vi "PD_Control.vi"() -> ()   [LabVIEW 2017]
uses:
  <vilib>/Platform/TimedLoop/XDataNode/timing_clust.ctl
  <vilib>/Platform/TimedLoop/XDataNode/nitl_modes.ctl
  <vilib>/Platform/TimedLoop/XDataNode/wakeup.ctl
  <vilib>/myRIO/Instrument Drivers/Onboard IO/AO/typedefs/AO Reference.ctl
  <vilib>/myRIO/Common/Instrument Driver Framework/Utilities/typedefs/myRIO Generic Hardware Reference.ctl
  <vilib>/myRIO/Common/Instrument Driver Framework/Utilities/typedefs/Hardware Version Enum.ctl
  <vilib>/myRIO/Common/Instrument Driver Framework/Utilities/typedefs/myRIO v1.0 Reference.ctl
  <vilib>/myRIO/Common/Instrument Driver Framework/Utilities/typedefs/Generic FPGA Reference.ctl
  <vilib>/myRIO/Common/Instrument Driver Framework/myRIO v1.0/AO/typedefs/AO Channels List.ctl
  <vilib>/myRIO/Common/Instrument Driver Framework/myRIO v1.0/AO/typedefs/AO Channels Enum.ctl
  <vilib>/myRIO/Common/Instrument Driver Framework/Utilities/typedefs/Analog Scaling Constants List.ctl
  <vilib>/myRIO/Common/Instrument Driver Framework/Utilities/typedefs/Analog Scaling Constants.ctl
  <vilib>/userdefined/High Color/nirio_resource_hc.ctl
  <vilib>/myRIO/Common/Instrument Driver Framework/Utilities/vis/Is FPGA Ref Available.vi
  <vilib>/myRIO/Common/Instrument Driver Framework/myRIO v1.0/AO/vis/myRIO v1.1 Open AO.vi
  <vilib>/myRIO/Instrument Drivers/Onboard IO/AO/vis/Write.vi
  <vilib>/myRIO/Common/Instrument Driver Framework/Utilities/vis/Validate Channels.vi
  <vilib>/myRIO/Common/Instrument Driver Framework/myRIO v1.0/AO/vis/myRIO v1.0 Reserve AO.vi
  <vilib>/myRIO/Common/Instrument Driver Framework/myRIO v1.0/AO/vis/myRIO v1.0 Build MUX Configuration AO.vi
  <vilib>/myRIO/Common/Instrument Driver Framework/myRIO v1.0/Resource Manager/vis/myRIO v1.0 Reserve Channel List.vi
  <vilib>/myRIO/Common/Instrument Driver Framework/myRIO v1.0/Resource Manager/vis/myRIO v1.0 Reserve Channel.vi
  <vilib>/myRIO/Common/Instrument Driver Framework/myRIO v1.0/Resource Manager/vis/myRIO v1.0 Unreserve Channel.vi
  <vilib>/myRIO/Common/Instrument Driver Framework/myRIO v1.0/Resource Manager/vis/myRIO v1.0 Build Mutex Name.vi
  <vilib>/Utility/VariantDataType/GetNumericInfo.vi
  <vilib>/Utility/error.llb/Error Cluster From Error Code.vi
  <vilib>/myRIO/Common/Instrument Driver Framework/myRIO v1.0/myRIO v1.1 Open.vi
  <vilib>/myRIO/Common/Instrument Driver Framework/myRIO v1.0/AO/vis/myRIO v1.0 Get Scaling Constants AO.vi
  <vilib>/myRIO/Common/Instrument Driver Framework/Utilities/vis/IO Manager.vi
  <vilib>/myRIO/Common/Instrument Driver Framework/Utilities/vis/Configuration Manager.vi
  <vilib>/myRIO/Common/Instrument Driver Framework/myRIO v1.0/myRIO v1.0 Close.vi
  <vilib>/myRIO/Common/Instrument Driver Framework/myRIO v1.0/AO/vis/myRIO v1.0 Write AO.vi
  <vilib>/addons/control/pid/pid.llb/PID (DBL).vi
  <vilib>/platform/TimedLoop/XDataNode/XDataNode.xnode
  <vilib>/myRIO/Express VI/Onboard IO/AO/AO Express VI.xnode
  <vilib>/myRIO/Instrument Drivers/Onboard IO/AO/vis/myRIO AO Open.xnode
  <vilib>/addons/control/pid/NI_PID_pid.lvlib
  <vilib>/myRIO/Instrument Drivers/Onboard IO/AO/AO.lvlib
  <vilib>/Platform/TimedLoop/XDataNode/XDNodeRunTimeDep.lvlib
panel:
  out "error out":errorcluster
  out "process variable":dbl
  out "Setpoint":dbl
  out "Analog Output":dbl(graph)=3.193359702
  out "output":dbl format="%.2f"
  in  "PID Range":cluster{"output high":dbl, "output low":dbl}={"output high"=3.2, "output low"=1.8} {"output low" format="%.2f"; "output high" format="%.2f"}
  in  "PID gains":T1={"proportional gain (Kc)"=2.0, "integral time (Ti, min)"=0.05, "derivative time (Td, min)"=0.0} {"derivative time (Td, min)" format="%.3f"; "integral time (Ti, min)" format="%.3f"; "proportional gain (Kc)" format="%.3f"}
  out "Distance":cluster{"setpoint":dbl, dbl}(graph)={"setpoint"=303.908879655711, 0.0}
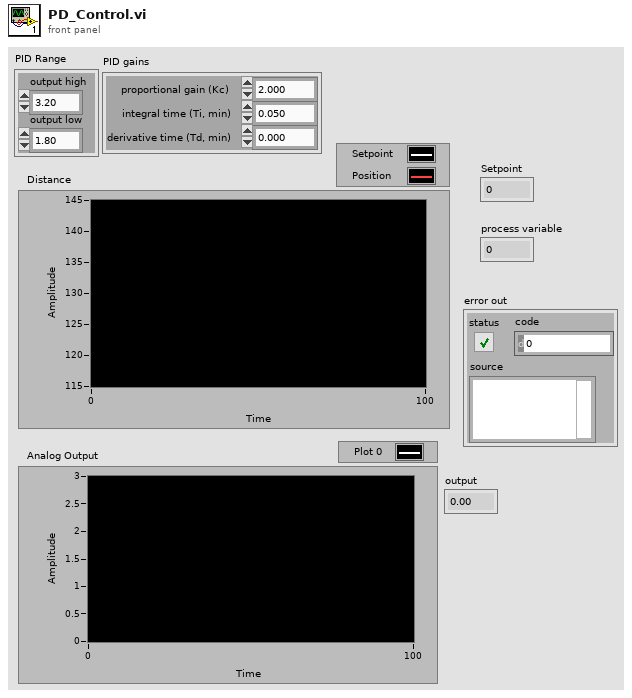
[diagram p1: front panel]
types:
  T1 = cluster{"proportional gain (Kc)":dbl, "integral time (Ti, min)":dbl, "derivative time (Td, min)":dbl}
  T2 = typedef "AO.lvlib/AO Reference.ctl" = cluster{"myRIO Reference":T3, "AO Channel List":T7, "AO Scaling Constant List":T9}
  T3 = typedef "myRIO Generic Hardware Reference.ctl" = cluster{"myRIO Model":T4, "myRIO Hardware Reference":T5}
  T4 = typedef "Hardware Version Enum.ctl" = enum16{"Unknown", "myRIO-1900", "myRIO-1950", "roboRIO", "NI ELVIS RIO CM"}
  T5 = typedef "myRIO v1.0 Reference.ctl" = cluster{"Generic FPGA Reference":T6, "Allow multiple opens":bool}
  T6 = typedef "Generic FPGA Reference.ctl" = refnum<k20>
  T7 = typedef "AO Channels List.ctl" = T8[]
  T8 = typedef "AO Channels Enum.ctl" = enum16{"Not Connected", "AudioOut/Left", "AudioOut/Right", "C/AO0", "C/AO1", "A/AO0", "A/AO1", "B/AO0", "B/AO1"}
  T9 = typedef "Analog Scaling Constants List.ctl" = T10[]
  T10 = typedef "Analog Scaling Constants.ctl" = cluster{"LSB Weight (Volts)":dbl, "Offset (Volts)":dbl, "Signed?":bool}
  T11 = typedef "nirio_resource_hc.ctl" = tag
  T12 = typedef "XDNodeRunTimeDep.lvlib/timing_clust.ctl" = cluster{"Expected End [f-1]":u64, "Actual End [f-1]":u64, "Finished Late? [f-1]":bool, "Expected End [i-1]":u64, "Actual End [i-1]":u64, "Finished Late? [i-1]":bool, "Expected Start [i]":u64, "Actual Start [i]":u64, "Expected Start [f]":u64, "Actual Start [f]":u64, "Source Name":string, "Structure Name":string, "Period":i64, "Deadline":i64, "Offset":i64, "Start":i64, "Priority":i32, "Timeout":i32, "Mode":T13, "Wakeup Reason":T14, "Error":errorcluster, "Source Type":string, "Secondary Source Type":string, "Global End Time":u64, "Global Start Time":u64, "Frame Duration":u64, "Iteration Duration":u64, "Assigned CPU":i32, "I/O Scan Engine Mode":u32}
  T13 = typedef "XDNodeRunTimeDep.lvlib/nitl_modes.ctl" = enum32{"No Change", "Process missed periods, maintain original phase", "Discard missed periods, maintain original phase", "Process missed periods, ignore original phase", "Discard missed periods, ignore original phase"}
  T14 = typedef "XDNodeRunTimeDep.lvlib/wakeup.ctl" = enum32{"Normal", "Aborted", "Asynchronous wakeup", "Timing source error", "Timed loop error", "Timeout"}
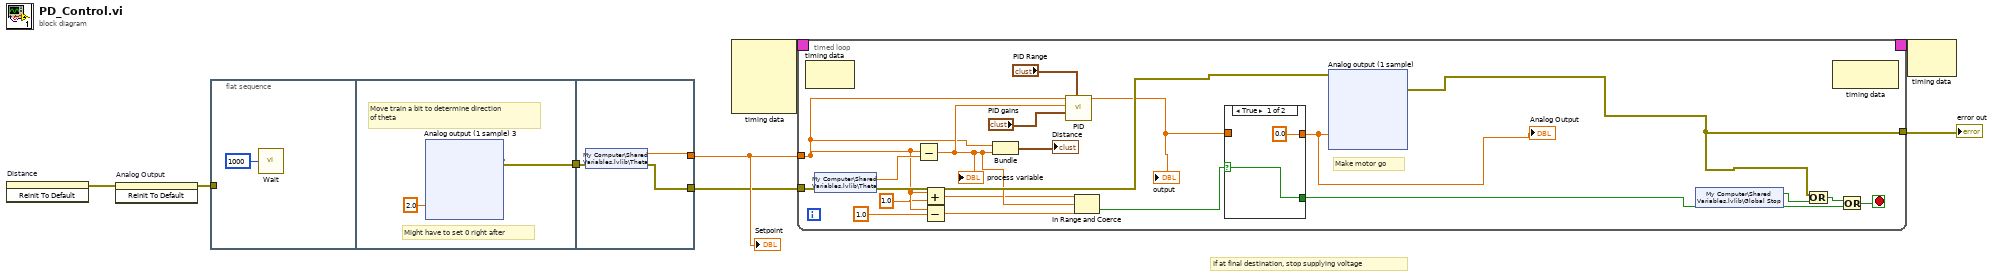
[diagram p0: block diagram]
diagram:
  # "If at final destination, stop supplying voltage"
  n1 = invoke on="Distance" class="WFChart (strict)" method="Reinit To Default"() -> (error out=w2:errorcluster)  [unwired: 3 in, 2 out]
  n2 = invoke on="Analog Output" class="WFChart (strict)" method="Reinit To Default"(error in=w2) -> (error out=w1:errorcluster)  [unwired: 2 in, 2 out]
  n3 = flat-sequence {
    tunnel: w1 -> [_]
    tunnel: [w10] -> w3
    tunnel: [w51] -> w6
    tunnel: [w50] -> w5
    tunnel: w3 -> [w49]
    frame #0 {
      n4 = call "Wait"("Count(mSec)"=u32 1000) -> ()  [unwired: 1 out]
    }
    frame #1 {
      # "Might have to set 0 right after"
      # "Move train a bit to determine direction\nof theta"
      n5 = xnode "Analog output (1 sample) 3"("C/AO0 (AO0)"=2.0) -> ("error out"=w10:errorcluster)  [unwired: 1 in]
    }
    frame #2 {
      n6 = shared-variable "My Computer\\Shared Variables.lvlib\\Theta"(error in=w49) -> (w51:dbl, error out=w50:errorcluster)
    }
  }
  n7 = node-c288() -> (w8:T12)  [unwired: 4 in]
  n8 = timed-loop {
    timing: w8 -> [_]
    timing-out: [_] -> w7
    tunnel: w6 -> [w64]
    tunnel: w5 -> [w68]
    tunnel: [w52] -> w4
    stop <- w54 stop-if-true
    # "Make motor go"
    n9 = node-c288() -> ()  [unwired: 1 in, 1 out]
    n10 = shared-variable "My Computer\\Shared Variables.lvlib\\Theta"(error in=w68) -> (w66:dbl, error out=w67:errorcluster)
    n11 = Subtract(x=w64, y=w66) -> (x-y=w65:dbl)
    "process variable" <- w65
    n12 = Add(x=w64, y=1.0) -> (x+y=w61:dbl)
    n13 = Subtract(x=w64, y=1.0) -> (x-y=w60:dbl)
    n14 = Bundle("Double"=w64, w65) -> (→"Distance":cluster{"Double":dbl, dbl})  [unwired: 1 in]
    n15 = call-poly <vilib>:"PID.vi"("output range"="PID Range", "PID gains"="PID gains", "process variable"=w65, "setpoint"=w64) -> ("output"=w58:dbl)  [unwired: 6 in, 1 out]
    "output" <- w58
    n16 = In Range and Coerce(upper limit=w61, x=w65, lower limit=w60) -> (In Range?=w59:bool)  [unwired: 1 out]
    n17 = case shown="True" w59 {
      selector: w59 -> [w72 w74]
      tunnel: [0.0 ("output") w75] -> w57
      tunnel: w58 -> [_ w75]
      tunnel: [w72 w74] -> w56
      frame True {
      }
      frame False {
      }
    }
    "Analog Output" <- w57
    n18 = xnode "Analog output (1 sample)"("C/AO0 (AO0)"=w57, "error in (no error)"=w67) -> ("error out"=w52:errorcluster)
    n19 = shared-variable "My Computer\\Shared Variables.lvlib\\Global Stop"() -> (w53:bool)  [unwired: 1 in, 1 out]
    n20 = Or(x=w52, y=w53) -> (x .or. y?=w55:bool)
    n21 = node-c288() -> ()  [unwired: 1 in, 1 out]
    n22 = Or(x=w55, y=w56) -> (x .or. y?=w54:bool)
  }
  "error out" <- w4
  n23 = node-c288(w7) -> ()  [unwired: 1 out]
  "Setpoint" <- w6
